vi "2d Gaussian array.vi"() -> (3 "Intensity Graph":u16[][](graph))   [LabVIEW 2020]
uses:
  NI_PtbyPt.lvlib
panel:
  out "Numeric 2":i32
  out "Numeric":i32
  in  "only noise":bool
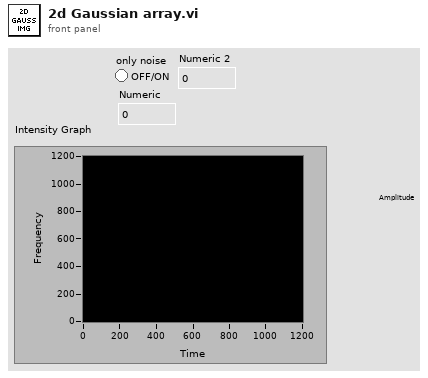
[diagram p1: front panel]
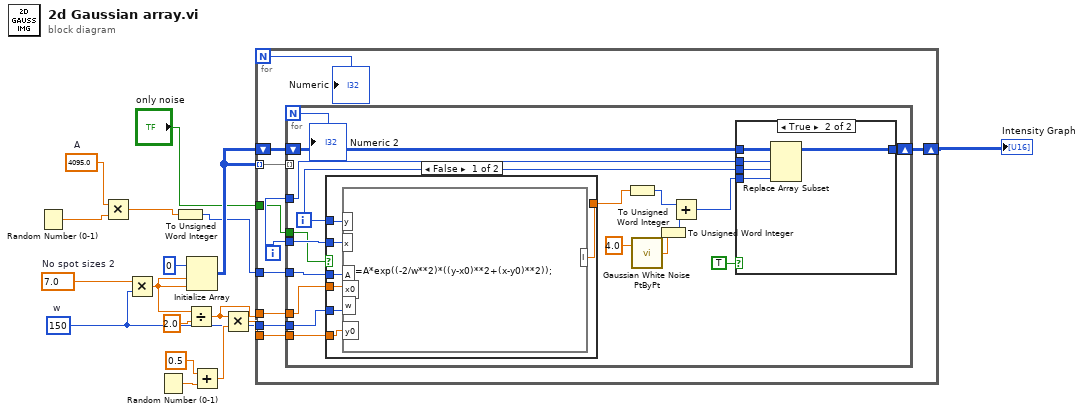
[diagram p0: block diagram]
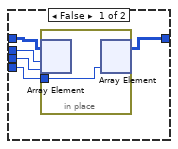
[diagram p2: hidden frame]
diagram:
  w17 = 4095.0  # A
  w8 = 7.0  # No spot sizes 2
  w9 = u8 150  # w
  n1 = Random Number (0-1)() -> (number: 0 to 1=w1:dbl)
  n2 = Multiply(x=w17, y=w1) -> (x*y=w4:dbl)
  n3 = Multiply(x=w8, y=w9) -> (x*y=w7:dbl)
  n4 = Random Number (0-1)() -> (number: 0 to 1=w12:dbl)
  n5 = To Unsigned Word Integer(number=w4) -> (unsigned 16bit integer=w3:u16)
  n6 = Divide(x=w7, y=2.0) -> (x/y=w15:dbl)
  n7 = Initialize Array(u16 0 ("element"), w7, w7) -> (w10:u16[][])
  n8 = Add(x=0.5, y=w12) -> (x+y=w14:dbl)
  n9 = Multiply(x=w15, y=w14) -> (x*y=w16:dbl)
  n10 = for {
    N -> [w18]
    tunnel: w10 -> [w27] mode=indexing
    shift-right: [w25] -> w5
    shift-left: w10 -> [w26]
    tunnel: w3 -> [w24]
    tunnel: w15 -> [w22]
    tunnel: w9 -> [w21]
    tunnel: w16 -> [w20]
    tunnel: "only noise" -> [w19]
    i -> [w23]
    n11 = for {
      N -> [w32]
      tunnel: w27 -> [_] mode=indexing
      shift-right: [w44] -> w25
      shift-left: w26 -> [w45]
      tunnel: w23 -> [w43]
      tunnel: w24 -> [w41]
      tunnel: w23 -> [w40]
      tunnel: w22 -> [w39]
      tunnel: w21 -> [w38]
      tunnel: w20 -> [w37]
      tunnel: w19 -> [w33]
      i -> [w42]
      n12 = case shown="False" w33 {
        tunnel: w42 -> [w63 _]
        tunnel: w41 -> [w62 _]
        tunnel: w40 -> [w61 _]
        tunnel: w39 -> [w60 _]
        tunnel: w38 -> [w59 _]
        tunnel: w37 -> [w58 _]
        tunnel: [w57 _] -> w29
        frame False {
          n13 = formula code="I=A*exp((-2/w**2)*((y-x0)**2+(x-y0)**2));"("y"=w63, "A"=w62, "x0"=w60, "x"=w61, "w"=w59, "y0"=w58) -> ("I"=w57:dbl)
        }
        frame True {
        }
      }
      n14 = To Unsigned Word Integer(number=w29) -> (unsigned 16bit integer=w28:u16)
      n15 = call "Gaussian White Noise PtByPt.vi"("standard deviation"=4.0) -> ("Gaussian white noise"=w35:dbl)  [unwired: 2 in]
      n16 = To Unsigned Word Integer(number=w35) -> (unsigned 16bit integer=w30:u16)
      n17 = Add(x=w28, y=w30) -> (x+y=w34:u16)
      n18 = case shown="True" TRUE {
        tunnel: w45 -> [w50 w56]
        tunnel: [w49 w55] -> w44
        tunnel: w43 -> [w48 w54]
        tunnel: w42 -> [w47 w53]
        tunnel: w34 -> [w46 w52]
        frame False {
          n19 = in-place {
            in-place-border: w46 -> [w51]
            n20 = in-place-array #1(w50, w48, w47) -> ()  [unwired: 1 out]
            n21 = in-place-array #1(w51) -> (w49:u16[][])  [unwired: 2 out]
          }
        }
        frame True {
          n22 = Replace Array Subset(array=w56, new element=w52, index (row)=w54, index (col)=w53) -> (w55:u16[][])
        }
      }
      "Numeric 2" <- w32
    }
    "Numeric" <- w18
  }
  "Intensity Graph" <- w5
